vi "niRFUtil WFM Complex Differential (complex array).vi"(7 "Complex Array In":T1 format="%.2f") -> (8 "Complex Array Out":T1 format="%.2f")   [LabVIEW 2015, in "niRFUtil.lvlib"]
doc: "(c) Copyright 2006, National Instruments, Inc. This VI may not be duplicated, sold, or distributed without written consent from National Instruments."
uses:
  niRFUtil.lvlib
  Includes/niRFUtil INC Complex Array.ctl
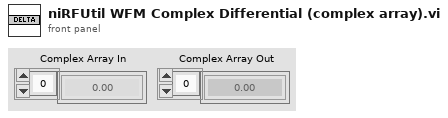
[diagram p1: front panel]
types:
  T1 = typedef "niRFUtil.lvlib/niRFUtil INC Complex Array.ctl" = csg[]
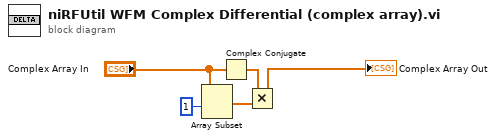
[diagram p0: block diagram]
diagram:
  n1 = Array Subset(array="Complex Array In", index=1) -> (w4:T1)  [unwired: 1 in]
  n2 = Complex Conjugate(1:"Complex Array In") -> (0:w3:T1)
  n3 = Multiply(x=w3, y=w4) -> (x*y=→"Complex Array Out":T1)
